vi "Check Unbundler.vi"(8 "error in (no error)":errorcluster, 10 "Bundler":refnum<vi>, 11 "Search in":refnum<class "Search.lvclass">) -> (0 "error out":errorcluster, 2 "Match?":bool, 3 "Search out":refnum<class "Search.lvclass">)   [LabVIEW 2016, in "Better Search.lvlib" / "Search.lvclass"]
uses:
  Search.lvclass
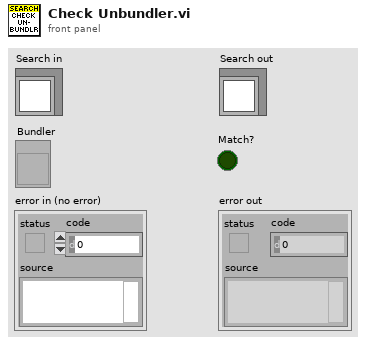
[diagram p1: front panel]
types:
  T1 = typedef "Better Search.lvlib/Search Type.ctl" = enum16{"Generic", "Text", "Data Type", "VI", "Node"}
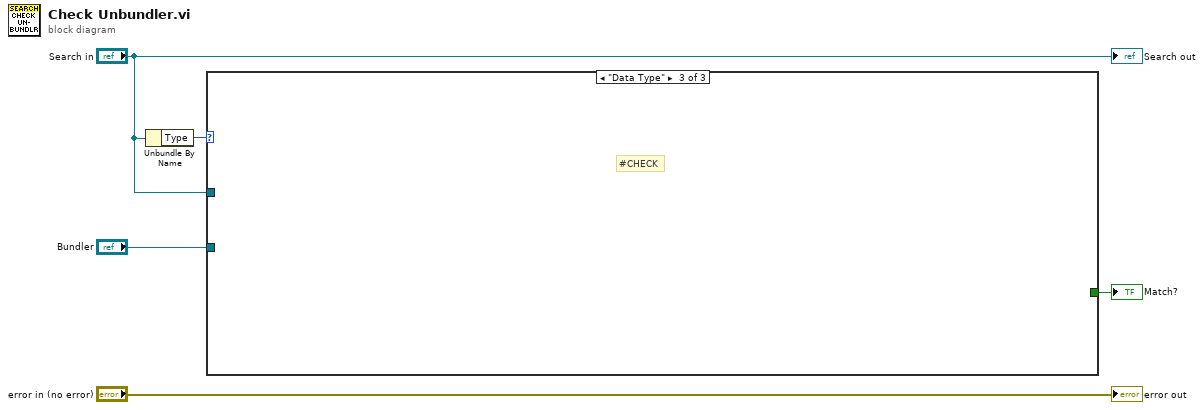
[diagram p0: block diagram]
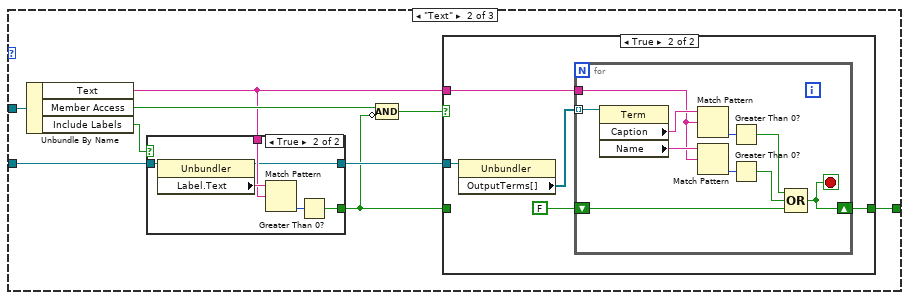
[diagram p3: hidden frame]
diagram:
  n1 = Unbundle By Name("Search in") -> ("Type"=w4:T1)
  n2 = case shown="\"Data Type\"" w4 {
    tunnel: "Search in" -> [_ w14 _]
    tunnel: [_ w12 _] -> w2
    tunnel: "Bundler" -> [_ w9 _]
    frame Default {
    }
    frame "Text" {
      n3 = Unbundle By Name(w14) -> ("Text"=w11:string, "Member Access"=w13:bool, "Include Labels"=w8:bool)
      n4 = case shown="True" w8 {
        tunnel: w11 -> [_ w19]
        tunnel: [w15 w18] -> w10
        tunnel: w9 -> [w15 w17]
        tunnel: [_ w16] -> w6
        frame False {
        }
        frame True {
          n5 = property class="Unbundler"(reference=w17) -> (reference out=w18:refnum<vi>, "Label.Text"=w20:string)  [unwired: 1 in, 1 out]
          n6 = Match Pattern(string=w20, regular expression=w19) -> (offset past match=w21:i32)  [unwired: 1 in, 3 out]
          n7 = Greater Than 0?(x=w21) -> (x > 0?=w16:bool)
        }
      }
      n8 = Compound Arithmetic op=AND(w13, invert w6) -> (w7:bool)
      n9 = case shown="True" w7 {
        tunnel: w11 -> [_ w27]
        tunnel: [w22 w25] -> w12
        tunnel: w10 -> [_ w23]
        tunnel: w6 -> [w22 _]
        frame False {
        }
        frame True {
          n10 = property class="Unbundler"(reference=w23) -> ("OutputTerms[]"=w24:refnum<vi>[])  [unwired: 1 in, 2 out]
          n11 = for {
            tunnel: w24 -> [w37] mode=indexing
            tunnel: w27 -> [w34]
            shift-right: [w28] -> w25
            shift-left: FALSE -> [w33]
            stop <- w28 stop-if-true
            n12 = property class="Term"(reference=w37) -> ("Caption"=w36:string, "Name"=w35:string)  [unwired: 1 in, 2 out]
            n13 = Match Pattern(string=w36, regular expression=w34) -> (offset past match=w31:i32)  [unwired: 1 in, 3 out]
            n14 = Match Pattern(string=w35, regular expression=w34) -> (offset past match=w32:i32)  [unwired: 1 in, 3 out]
            n15 = Greater Than 0?(x=w31) -> (x > 0?=w30:bool)
            n16 = Greater Than 0?(x=w32) -> (x > 0?=w29:bool)
            n17 = Compound Arithmetic op=OR(w30, w29, w33) -> (w28:bool)
          }
        }
      }
    }
    frame "Data Type" {
      # "#CHECK"
    }
  }
  "Match?" <- w2
  "error out" <- "error in (no error)"
  "Search out" <- "Search in"
